vi "Service Mode Test Select.vi"(0 "GEA2 Reference In":refnum<k24>, 5 "High\\Low End":enum16{"HE", "LE"}(ring), 7 "Test Number":T1=enum."Test 1 - Fault Codes", 11 "Error In":errorcluster) -> (4 "GEA2 Reference Out":refnum<k24>, 15 "Error Out":errorcluster)   [LabVIEW 2016, in "TLMB.lvlib"]
uses:
  Projects/TLMB.lvlib
  Q:/Common/DLLs/GEA3/GeaCommunication.dll
  Common/DLLs/GEA3/GeaCommunication.dll
  type defs/Service mode Tests.ctl
  Common/LabVIEW GEA2 Toolkit/LabVIEW_GEA2_Toolkit.lvlibp/type defs/Source_Destination.ctl
  Common/LabVIEW GEA2 Toolkit/LabVIEW_GEA2_Toolkit.lvlibp/type defs/ERD Write Data In.ctl
  Common/LabVIEW GEA2 Toolkit/LabVIEW_GEA2_Toolkit.lvlibp/type defs/Data Type.ctl
  Common/LabVIEW GEA2 Toolkit/LabVIEW_GEA2_Toolkit.lvlibp
panel:
  in  "Standalone?":bool
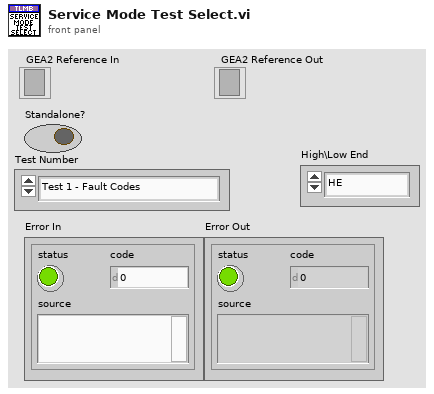
[diagram p1: front panel]
types:
  T1 = typedef "TLMB.lvlib/Service mode Tests.ctl" = enum16{"Test 0 - All LEDs on", "Test 1 - Fault Codes", "Test 2 - Personality ID", "Test 3 - UI Software Ver(Crit)", "Test 4 - UI Software Ver(Non-crit)", "Test 5 - XML Ver (Non-Crit) ", "Test 6 - Hot Water Valve", "Test 7 - Cold Water Valve", "Test 8 - Fabric Softener Disp", "Test 9 - Spray Rinse Valve Check", "Test 10 - Pressure Sensor", "Test 11 - Recirc Pump", "Test 12 - Drain Pump", "Test 13 - Lid Switch", "Test 14 - Spin", "Test 15 - Agitate", "Test 16 - Clear all Fcodes", "Test 17 - Change Personality", "Test 18 - Analog Knob"}
  T2 = typedef "LabVIEW_GEA2_Toolkit.lvlibp/ERD Write Data In.ctl" = cluster{"ERD Number":u16, "Data Type":T3, "Data":string}
  T3 = typedef "LabVIEW_GEA2_Toolkit.lvlibp/Data Type.ctl" = enum16{"string", "boolean", "uint8_t", "uint16_t", "uint32_t", "uint64_t", "int8_t", "int16_t", "int32_t", "int64_t"}
  T4 = typedef "LabVIEW_GEA2_Toolkit.lvlibp/Source_Destination.ctl" = cluster{"Source":u8, "Destination":u8}
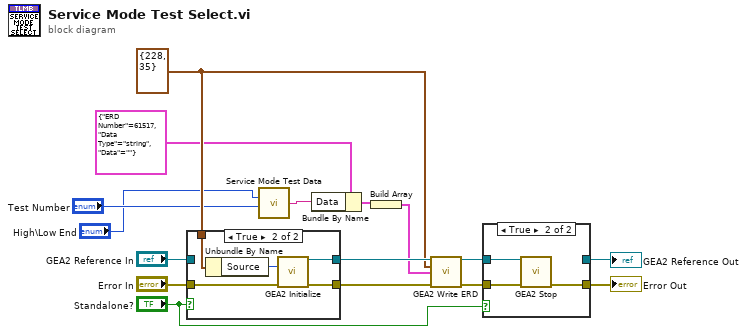
[diagram p0: block diagram]
diagram:
  w6 = T4 {"Source"=228, "Destination"=35} ("GEA Inputs")
  n1 = case shown="True" "Standalone?" {
    tunnel: "Error In" -> [w17 w23]
    tunnel: [w17 w22] -> w11
    tunnel: "GEA2 Reference In" -> [w18 _]
    tunnel: [w18 w21] -> w9
    tunnel: w6 -> [_ w19]
    frame False {
    }
    frame True {
      n2 = Unbundle By Name(w19) -> ("Source"=w20:u8)
      n3 = call "GEA2 Initialize.vi"("Source Address"=w20, "error in"=w23) -> ("GEA2 Reference Out"=w21:refnum<k24>, "error out"=w22:errorcluster)  [unwired: 11 in, 1 out]
    }
  }
  n4 = call "Service Mode Test Data.vi"("High\\Low End"="High\\Low End", "Switch"="Test Number") -> ("Switch Message"=w3:string)  [unwired: 13 in]
  n5 = Bundle By Name(cluster=T2 {"ERD Number"=61517, "Data Type"=enum."string", "Data"=""} ("ERD Write Data In"), "Data"=w3) -> (w8:T2)
  n6 = Build Array(w8) -> (w7:T2[])
  n7 = call "GEA2 Write ERD.vi"("GEA2 Reference In"=w9, "GEA Inputs"=w6, "Write ERD List"=w7, "Error In"=w11) -> ("GEA2 Reference Out"=w5:refnum<k24>, "Error Out"=w10:errorcluster)  [unwired: 9 in, 1 out]
  n8 = case shown="True" "Standalone?" {
    tunnel: [w24 w28] -> w14
    tunnel: w5 -> [w25 w27]
    tunnel: [w25 _] -> w13
    tunnel: w10 -> [w24 w26]
    frame False {
    }
    frame True {
      n9 = call "GEA2 Stop.vi"("GEA2 Reference In"=w27, "Error In"=w26) -> ("Error Out"=w28:errorcluster)  [unwired: 13 in]
    }
  }
  "Error Out" <- w14
  "GEA2 Reference Out" <- w13
